vi "TestPumps.vi"(11 "Stand in":refnum<class "Stand.lvclass">) -> (3 "Stand out":refnum<class "Stand.lvclass">)   [LabVIEW 2019, in "Stand.lvclass"]
uses:
  Stand.lvclass
  Stand.lvclass/Stand.ctl
  Engine_1DI_2DO_class/Engine_1DI_2DO.lvclass
panel:
  in  "TurnOff":bool
  in  "TurnOn":bool
  in  "index":i32
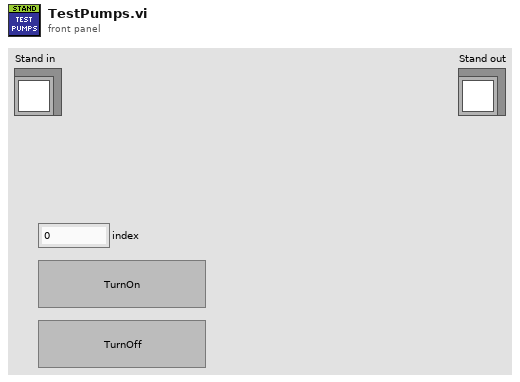
[diagram p1: front panel]
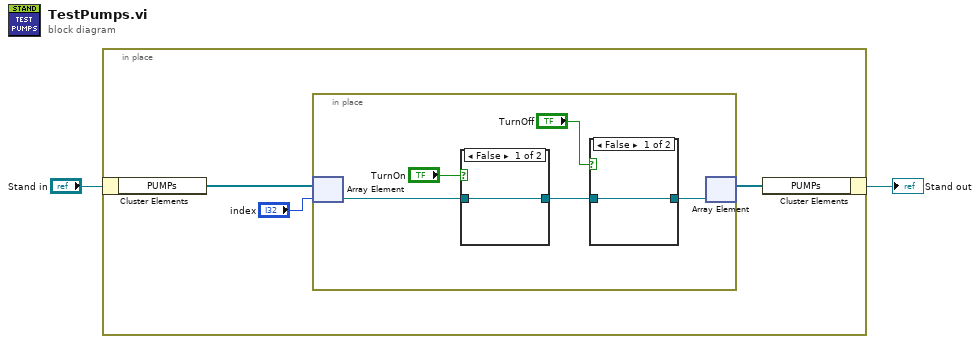
[diagram p0: block diagram]
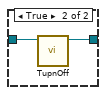
[diagram p2: hidden frame]
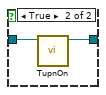
[diagram p3: hidden frame]
diagram:
  n1 = in-place {
    n2 = in-place-cluster #1("Stand in") -> ("PUMPs"=w5:refnum<class "Engine_1DI_2DO.lvclass">[])
    n3 = in-place {
      n4 = in-place-array #2(w5, "index") -> (w10:refnum<class "Engine_1DI_2DO.lvclass">)
      n5 = case shown="False" "TurnOn" {
        tunnel: w10 -> [w14 w16]
        tunnel: [w14 w15] -> w9
        frame False {
        }
        frame True {
          n6 = call "TupnOn.vi"("Pump_1AI_1DO_2DI in"=w16) -> ("Pump_1AI_1DO_2DI out"=w15:refnum<class "Engine_1DI_2DO.lvclass">)  [unwired: 10 in]
        }
      }
      n7 = case shown="False" "TurnOff" {
        tunnel: w9 -> [w11 w13]
        tunnel: [w11 w12] -> w8
        frame False {
        }
        frame True {
          n8 = call "TupnOff.vi"("Pump_1AI_1DO_2DI in"=w13) -> ("Pump_1AI_1DO_2DI out"=w12:refnum<class "Engine_1DI_2DO.lvclass">)  [unwired: 10 in]
        }
      }
      n9 = in-place-array #2(w8) -> (w3:refnum<class "Engine_1DI_2DO.lvclass">[])  [unwired: 1 out]
    }
    n10 = in-place-cluster #1("PUMPs"=w3) -> (→"Stand out":refnum<class "Stand.lvclass">)
  }
